vi "even with subvi.vi"() -> ()   [LabVIEW 2020]
panel:
  out "String 3":string
  in  "String 2":string
  in  "String":string
  in  "input":dbl
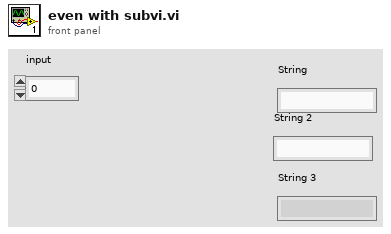
[diagram p1: front panel]
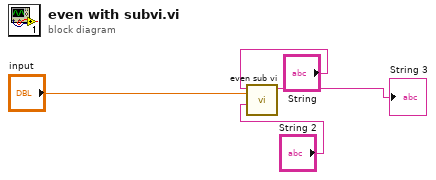
[diagram p0: block diagram]
diagram:
  n1 = call "even sub vi.vi"("String 2"="String 2", "input"="input", "String"="String") -> ("String 3"=→"String 3":string)  [unwired: 8 in]
